vi "Capture Background (SubVI).vi"(8 "Find Min":bool, 11 "Frame In":u8[][](array[numeric])) -> (2 "Background Captured":bool, 3 "BG Image":u8[][](array[numeric]))   [LabVIEW 2015]
panel:
  out "Count":u16
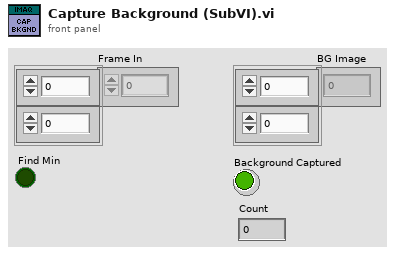
[diagram p1: front panel]
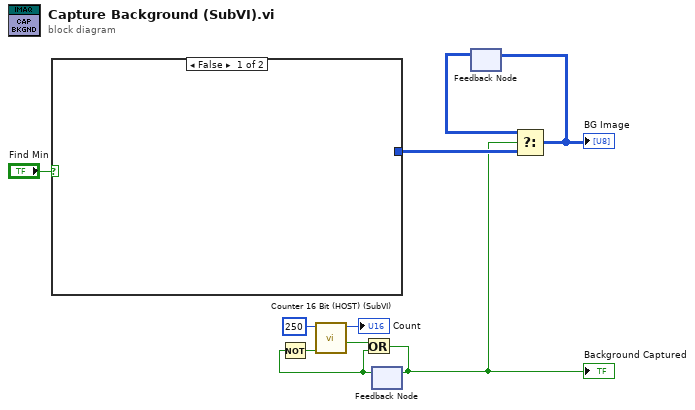
[diagram p0: block diagram]
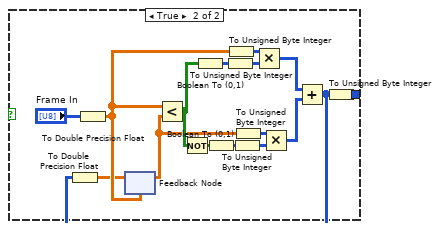
[diagram p2: hidden frame]
diagram:
  n1 = case shown="False" "Find Min" {
    tunnel: [_ w26] -> w10
    frame False {
    }
    frame True {
      n2 = To Double Precision Float(number="Frame In") -> (double precision float=w13:dbl[][])
      n3 = feedback #1(w13) -> (w16:dbl[][])
      n4 = Less?(x=w13, y=w16) -> (x < y?=w18:bool[][])
      n5 = Not(x=w18) -> (.not. x?=w17:bool[][])
      n6 = Boolean To (0,1)(Boolean=w18) -> (0, 1=w24:i16[][])
      n7 = Boolean To (0,1)(Boolean=w17) -> (0, 1=w19:i16[][])
      n8 = To Unsigned Byte Integer(number=w24) -> (unsigned 8bit integer=w22:u8[][])
      n9 = To Unsigned Byte Integer(number=w13) -> (unsigned 8bit integer=w23:u8[][])
      n10 = To Unsigned Byte Integer(number=w19) -> (unsigned 8bit integer=w21:u8[][])
      n11 = To Unsigned Byte Integer(number=w16) -> (unsigned 8bit integer=w20:u8[][])
      n12 = Multiply(x=w23, y=w22) -> (x*y=w15:u8[][])
      n13 = Multiply(x=w20, y=w21) -> (x*y=w14:u8[][])
      n14 = Add(x=w15, y=w14) -> (x+y=w11:u8[][])
      n15 = To Double Precision Float(number=w11) -> (double precision float=w12:dbl[][])
      n16 = feedback-in #1(w12) -> ()
      n17 = To Unsigned Byte Integer(number=w11) -> (unsigned 8bit integer=w26:u8[][])
    }
  }
  n18 = feedback #2() -> (w8:bool)  [unwired: 1 in]
  n19 = Not(x=w8) -> (.not. x?=w9:bool)
  n20 = call "Counter 16 Bit (HOST) (SubVI).vi"("Enable"=w9, "Max. Count"=u16 250) -> ("Count End?"=w7:bool, "Count"=→"Count":u16)  [unwired: 7 in, 1 out]
  n21 = Or(x=w7, y=w8) -> (x .or. y?=w4:bool)
  "Background Captured" <- w4
  n22 = feedback-in #2(w4) -> ()
  n23 = feedback #3() -> (w3:u8[][])  [unwired: 1 in]
  n24 = Select(t=w3, s=w4, f=w10) -> (s? t:f=w2:u8[][])
  "BG Image" <- w2
  n25 = feedback-in #3(w2) -> ()
